vi "SLL DE DO Engine.vi"(8 "error in (no error)":errorcluster) -> (0 "error out":errorcluster)   [LabVIEW 2009]
doc: "Copyright © 2005, Soliton Technologies.\nAll rights reserved."
uses:
  Controls/SLL DE DAQ Engine Options.ctl
  Controls/SLL DE DO Response LV2Global Options.ctl
  Controls/SLL DE DAQ Global Elements.ctl
  Controls/SLL DE DAQ Global Options.ctl
  Controls/SLL DE DO Global Options.ctl
  Controls/SLL DE DO Safe Value Global Options.ctl
  Controls/SLL DE DO Command LV2Global Options.ctl
  <vilib>/DAQmx/write.llb/DAQmx Write (Digital Bool 1Line 1Point).vi
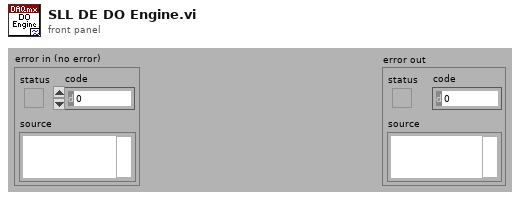
[diagram p1: front panel]
types:
  T1 = typedef "SLL DE DAQ Engine Options.ctl" = enum16{">Init", ">Safe Mode", ">Poll", ">Error", ">Exit", ">Restart", ">DI", ">DO", ">AI", ">AO", ">Start Task", ">Stop Task"}
  T2 = typedef "SLL DE DO Response LV2Global Options.ctl" = enum16{"Initialize", "Send Response", "Check Response", "Close"}
  T3 = cluster{"Previous DO Data":bool[], "Executed for":string, "DO Channels":refnum<k21>[]}
  T4 = typedef "SLL DE DAQ Global Elements.ctl" = enum16{"AI Error", "AO Error", "DI Error", "DO Error", "AI Restart", "DI Restart", "AI Running", "AO Running", "DI Running", "DO Running", "DAQ Exit?"}
  T5 = typedef "SLL DE DAQ Global Options.ctl" = enum16{"Init", "Write 1", "Read 1", "Write Array", "Read Array", "Clear"}
  T6 = typedef "SLL DE DO Global Options.ctl" = enum16{"Init", "Write Line", "Write Array", "Write Full Status", "Read Line", "Read Array", "Read Full Status", "Restart DO", "Send to Safe Mode", "Stop DO"}
  T7 = typedef "SLL DE DO Command LV2Global Options.ctl" = enum16{"Init/Register Events", "Get Event Refnum", "Fire Event", "Destroy Event"}
  T8 = typedef "SLL DE DO Safe Value Global Options.ctl" = enum16{"Read", "Write"}
  T9 = typedef "SLL DE List of Digital Outputs.ctl" = enum16{"STATION1_START TEST", "STATION1_STOP TEST", "STATION1_LIGHT1", "STATION1_LIGHT2", "STATION1_LIGHT3", "STATION2_START TEST", "STATION2_STOP TEST", "STATION2_LIGHT1", "STATION2_LIGHT2", "STATION2_LIGHT3", "STATION3_START TEST", "STATION3_STOP TEST", "STATION3_LIGHT1", "STATION3_LIGHT2", "STATION3_LIGHT3", "STATION4_START TEST", "STATION4_STOP TEST", "STATION4_LIGHT1", "STATION4_LIGHT2", "STATION4_LIGHT3"}
  T10 = enum16{"Left Button", "Center Button", "Right Button", "Window Close"}
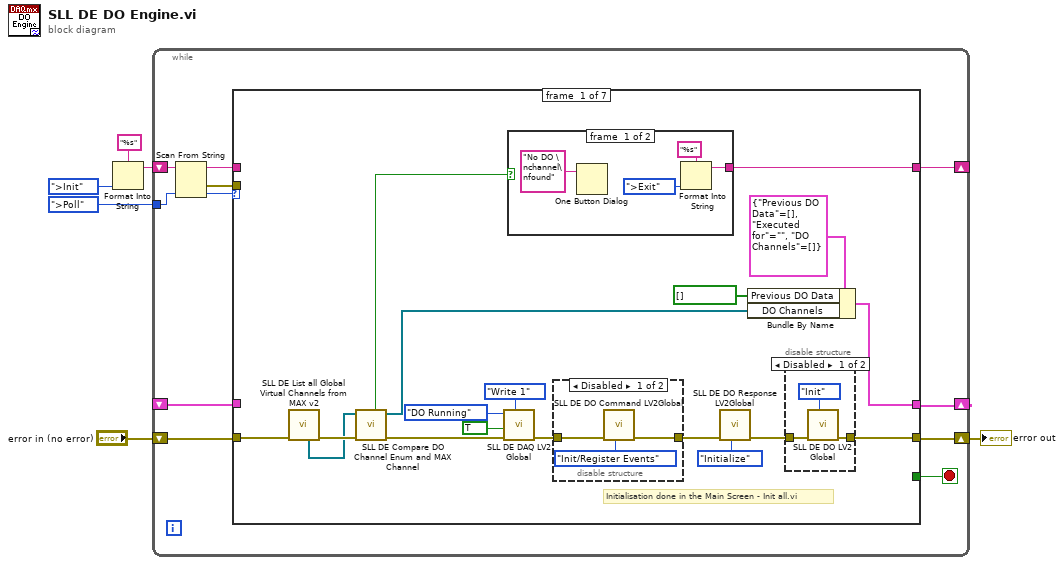
[diagram p0: block diagram]
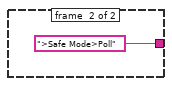
[diagram p4: hidden frame]
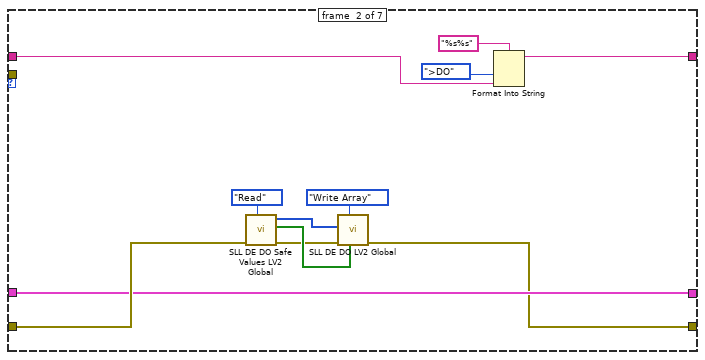
[diagram p5: hidden frame]
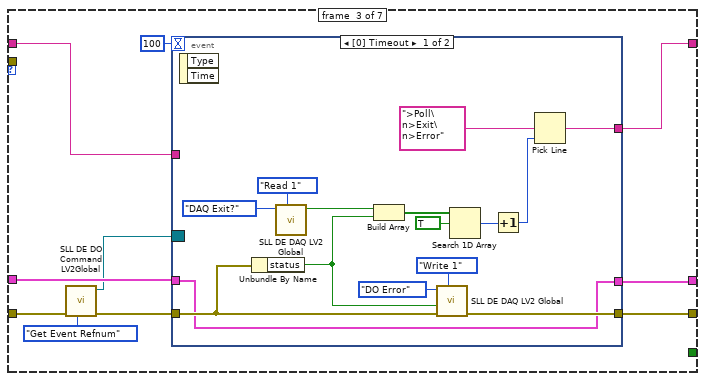
[diagram p6: hidden frame]
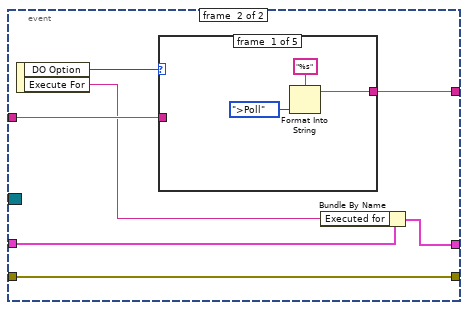
[diagram p7: hidden frame]
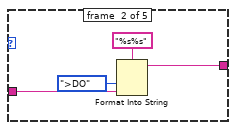
[diagram p8: hidden frame]
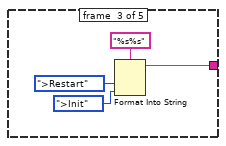
[diagram p9: hidden frame]
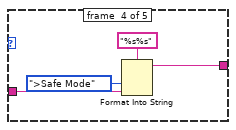
[diagram p10: hidden frame]
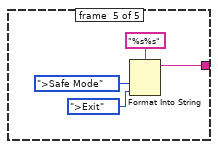
[diagram p11: hidden frame]
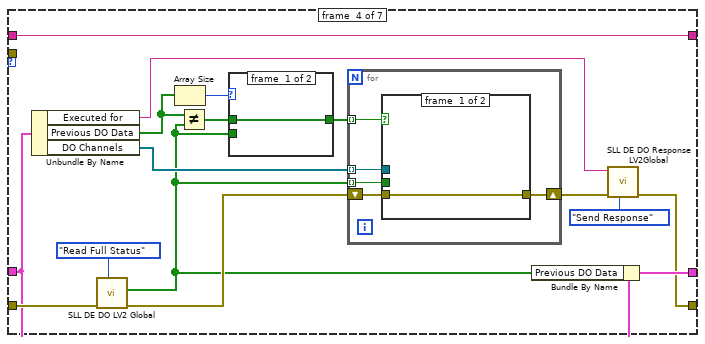
[diagram p12: hidden frame]
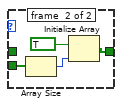
[diagram p13: hidden frame]
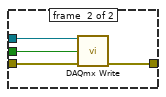
[diagram p14: hidden frame]
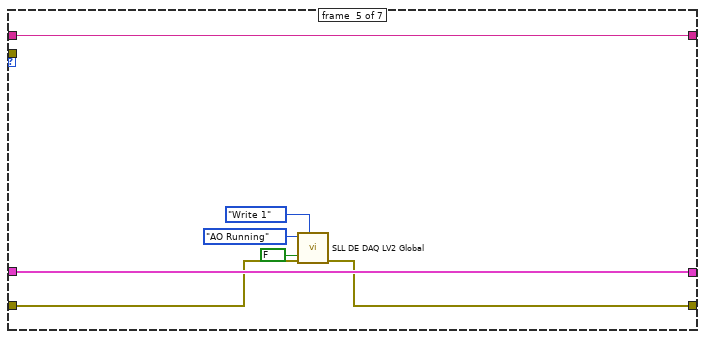
[diagram p15: hidden frame]
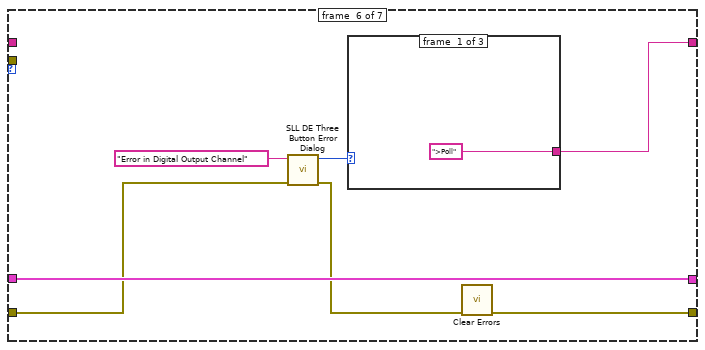
[diagram p16: hidden frame]
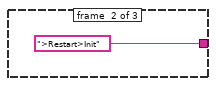
[diagram p17: hidden frame]
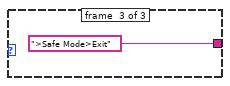
[diagram p18: hidden frame]
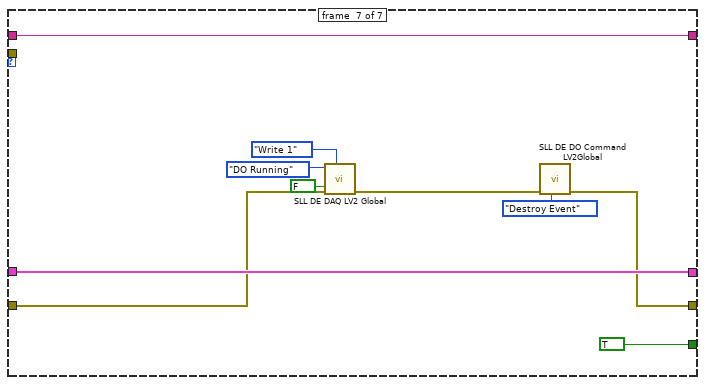
[diagram p19: hidden frame]
diagram:
  n1 = Format Into String(format string="%s", SLL_DE_DAQ_Engine_Options.">Init" ("DAQ Options")) -> (resulting string=w2:string)  [unwired: 2 in, 1 out]
  n2 = while {
    shift-right: [w16] -> w5
    shift-left: "error in (no error)" -> [w17]
    shift-right: [w15] -> _
    shift-left: _ -> [w14]
    shift-right: [w10] -> _
    shift-left: w2 -> [w13]
    tunnel: SLL_DE_DAQ_Engine_Options.">Poll" ("DAQ Options") -> [w7]
    stop <- w9 stop-if-true
    n3 = Scan From String(input string=w13, default 1=w7) -> (remaining string=w12:string, error out=w11:errorcluster, output 1=w8:T1)  [unwired: 3 in, 1 out]
    n4 = case shown="\">Safe Mode\"" w8 {
      tunnel: w17 -> [w28 w57 w67 w125 w144 w154 w163]
      tunnel: [w20 w49 w65 w115 w143 w150 w160] -> w16
      tunnel: [w34 w54 w64 w123 w149 w156 w169] -> w15
      tunnel: w14 -> [_ w54 w66 w112 w149 w156 w169]
      tunnel: w12 -> [_ w52 w62 w124 w148 _ w168]
      tunnel: w11 -> [_ _ _ _ _ _ _]
      tunnel: [w33 w51 w63 w124 w148 w152 w168] -> w10
      tunnel: [_ _ _ _ _ _ TRUE] -> w9
      frame #0 {
        # "Initialisation done in the Main Screen - Init all.vi"
        n5 = call "SLL DE List all Global Virtual Channels from MAX v2.vi"("error in (no error)"=w28) -> ("error out"=w29:errorcluster, "Digital Output"=w26:refnum<k21>[])  [unwired: 4 in, 5 out]
        n6 = call "SLL DE Compare DO Channel Enum and MAX Channel.vi"("error in (no error)"=w29, "Digital Output Channels"=w26) -> ("error out"=w25:errorcluster, "Channels Out"=w19:refnum<k21>[], "Pass?"=w27:bool)  [unwired: 7 in]
        n7 = call "SLL DE DAQ LV2 Global.vi"("Option"=SLL_DE_DAQ_Global_Options."Write 1", "error in (no error)"=w25, "Status In"=TRUE, "Element"=SLL_DE_DAQ_Global_Elements."DO Running") -> ("error out"=w24:errorcluster)  [unwired: 5 in, 2 out]
        n8 = case shown="False" w27 {
          tunnel: [w45 ">Safe Mode>Poll"] -> w33
          frame #0 {
            n9 = One Button Dialog(message="No DO \nchannel\nfound") -> ()  [unwired: 1 in, 1 out]
            n10 = Format Into String(format string="%s", SLL_DE_DAQ_Engine_Options.">Exit" ("DAQ Options")) -> (resulting string=w45:string)  [unwired: 2 in, 1 out]
          }
          frame #1 {
          }
        }
        n11 = disable-structure shown="Disabled" {
          disable-tunnel: w24 -> [w42 w43]
          disable-tunnel: [w40 w43] -> w23
          frame #0 {
            n12 = call "SLL DE DO Command LV2Global.vi"("Option"=SLL_DE_DO_Command_LV2Global_Options."Init/Register Events", "Error in (no error)"=w42) -> ("Error out"=w40:errorcluster)  [unwired: 8 in, 1 out]
          }
          frame #1 {
          }
        }
        n13 = call "SLL DE DO Response LV2Global.vi"("Option"=SLL_DE_DO_Response_LV2Global_Options."Initialize", "Error in (no error)"=w23) -> ("Error out"=w21:errorcluster)  [unwired: 8 in, 1 out]
        n14 = Bundle By Name(cluster=T3 {"Previous DO Data"=[], "Executed for"="", "DO Channels"=[]} ("Data Cluster"), "Previous DO Data"=bool[] [], "DO Channels"=w19) -> (w34:T3)
        n15 = disable-structure shown="Disabled" {
          disable-tunnel: w21 -> [w37 w39]
          disable-tunnel: [w36 w39] -> w20
          frame #0 {
            n16 = call "SLL DE DO LV2 Global.vi"("DO Option"=SLL_DE_DO_Global_Options."Init", "Error In"=w37) -> ("error out"=w36:errorcluster)  [unwired: 6 in, 3 out]
          }
          frame #1 {
          }
        }
      }
      frame #1 {
        n17 = call "SLL DE DO Safe Values LV2 Global.vi"("Cases"=SLL_DE_DO_Safe_Value_Global_Options."Read", "error in (no error)"=w57) -> ("error out"=w58:errorcluster, "Value Array Out"=w59:bool[], "Elements Out"=w60:T9[])  [unwired: 7 in]
        n18 = call "SLL DE DO LV2 Global.vi"("DO State Array"=w59, "DO Option"=SLL_DE_DO_Global_Options."Write Array", "Error In"=w58, "DO Channel Name Array"=w60) -> ("error out"=w49:errorcluster)  [unwired: 4 in, 3 out]
        n19 = Format Into String(format string="%s%s", SLL_DE_DAQ_Engine_Options.">DO" ("DAQ Options"), w52) -> (resulting string=w51:string)  [unwired: 2 in, 1 out]
      }
      frame #2 {
        n20 = call "SLL DE DO Command LV2Global.vi"("Option"=SLL_DE_DO_Command_LV2Global_Options."Get Event Refnum", "Error in (no error)"=w67) -> ("Error out"=w68:errorcluster, "Event Registration Refnum"=w61:refnum<event-registration>)  [unwired: 8 in]
        n21 = event shown="[0] Timeout" {
          selector: w61 -> [_ _]
          dyn-events: _ -> [_ _]
          timeout: 100 -> [_ _]
          tunnel: w68 -> [w76 w91]
          tunnel: [w77 w91] -> w65
          tunnel: [w75 w89] -> w63
          tunnel: w62 -> [_ w90]
          tunnel: w66 -> [w74 w88]
          tunnel: [w74 w86] -> w64
          event #0 {
            n22 = event-data() -> ()  [unwired: 1 in, 2 out]
            n23 = Unbundle By Name(w76) -> ("status"=w85:bool)
            n24 = call "SLL DE DAQ LV2 Global.vi"("Option"=SLL_DE_DAQ_Global_Options."Read 1", "Element"=SLL_DE_DAQ_Global_Elements."DAQ Exit?") -> ("Status Out"=w71:bool)  [unwired: 7 in, 2 out]
            n25 = Build Array(w71, w85) -> (w79:bool[])
            n26 = call "SLL DE DAQ LV2 Global.vi"("Option"=SLL_DE_DAQ_Global_Options."Write 1", "error in (no error)"=w76, "Status In"=w85, "Element"=SLL_DE_DAQ_Global_Elements."DO Error") -> ("error out"=w77:errorcluster)  [unwired: 5 in, 2 out]
            n27 = Search 1D Array(1D array=w79, element=TRUE) -> (index of element=w81:i32)  [unwired: 1 in]
            n28 = Increment(x=w81) -> (x+1=w82:i32)
            n29 = Pick Line(multi-line string=">Poll\n>Exit\n>Error", line index=w82) -> (output string=w75:string)  [unwired: 1 in]
          }
          event #1 {
            n30 = event-data() -> ("DO Option"=w92:T6, "Execute For"=w87:string)  [unwired: 1 in]
            n31 = case shown="\"Init\", Default" w92 {
              tunnel: w90 -> [_ w97 _ w105 _]
              tunnel: [w93 w96 w100 w104 w109] -> w89
              frame #0 {
                n32 = Format Into String(format string="%s", SLL_DE_DAQ_Engine_Options.">Poll" ("DAQ Options")) -> (resulting string=w93:string)  [unwired: 2 in, 1 out]
              }
              frame #1 {
                n33 = Format Into String(format string="%s%s", SLL_DE_DAQ_Engine_Options.">DO" ("DAQ Options"), w97) -> (resulting string=w96:string)  [unwired: 2 in, 1 out]
              }
              frame #2 {
                n34 = Format Into String(format string="%s%s", SLL_DE_DAQ_Engine_Options.">Restart" ("DAQ Options"), SLL_DE_DAQ_Engine_Options.">Init" ("DAQ Options")) -> (resulting string=w100:string)  [unwired: 2 in, 1 out]
              }
              frame #3 {
                n35 = Format Into String(format string="%s%s", SLL_DE_DAQ_Engine_Options.">Safe Mode" ("DAQ Options"), w105) -> (resulting string=w104:string)  [unwired: 2 in, 1 out]
              }
              frame #4 {
                n36 = Format Into String(format string="%s%s", SLL_DE_DAQ_Engine_Options.">Safe Mode" ("DAQ Options"), SLL_DE_DAQ_Engine_Options.">Exit" ("DAQ Options")) -> (resulting string=w109:string)  [unwired: 2 in, 1 out]
              }
            }
            n37 = Bundle By Name(cluster=w88, "Executed for"=w87) -> (w86:T3)
          }
        }
      }
      frame #3 {
        n38 = Unbundle By Name(w112) -> ("Executed for"=w113:string, "Previous DO Data"=w119:bool[], "DO Channels"=w120:refnum<k21>[])
        n39 = call "SLL DE DO LV2 Global.vi"("DO Option"=SLL_DE_DO_Global_Options."Read Full Status", "Error In"=w125) -> ("error out"=w126:errorcluster, "Digital Array Status"=w118:bool[])  [unwired: 6 in, 2 out]
        n40 = Array Size(array=w119) -> (size(s)=w122:i32)
        n41 = Not Equal?(x=w119, y=w118) -> (x != y?=w121:bool[])
        n42 = case shown="0" w122 {
          tunnel: w121 -> [w128 _]
          tunnel: [w128 w131] -> w117
          tunnel: w118 -> [_ w130]
          frame #0 {
          }
          frame #1 {
            n43 = Array Size(array=w130) -> (size(s)=w129:i32)
            n44 = Initialize Array(TRUE, w129) -> (w131:bool[])
          }
        }
        n45 = for {
          tunnel: w117 -> [w137] mode=indexing
          tunnel: w118 -> [w136] mode=indexing
          shift-right: [w134] -> w116
          shift-left: w126 -> [w135]
          tunnel: w120 -> [w133] mode=indexing
          n46 = case shown="True" w137 {
            tunnel: w136 -> [_ w142]
            tunnel: w135 -> [w138 w141]
            tunnel: [w138 w140] -> w134
            tunnel: w133 -> [_ w139]
            frame #0 {
            }
            frame #1 {
              n47 = call-poly <vilib>:"DAQmx Write.vi"("task/channels in"=w139, "data"=w142, "error in"=w141) -> ("error out"=w140:errorcluster)  [unwired: 10 in, 2 out]
            }
          }
        }
        n48 = Bundle By Name(cluster=w112, "Previous DO Data"=w118) -> (w123:T3)
        n49 = call "SLL DE DO Response LV2Global.vi"("Option"=SLL_DE_DO_Response_LV2Global_Options."Send Response", "Error in (no error)"=w116, "Executed For?"=w113) -> ("Error out"=w115:errorcluster)  [unwired: 7 in, 1 out]
      }
      frame #4 {
        n50 = call "SLL DE DAQ LV2 Global.vi"("Option"=SLL_DE_DAQ_Global_Options."Write 1", "error in (no error)"=w144, "Status In"=FALSE, "Element"=SLL_DE_DAQ_Global_Elements."AO Running") -> ("error out"=w143:errorcluster)  [unwired: 5 in, 2 out]
      }
      frame #5 {
        n51 = call "SLL DE Three Button Error Dialog.vi"("Error In"=w154, "Window Title"="Error in Digital Output Channel") -> ("Error Out"=w151:errorcluster, "Which Button?"=w153:T10)  [unwired: 8 in]
        n52 = case shown="\"Center Button\"" w153 {
          tunnel: [">Poll" ("Window Title") ">Restart>Init" ("Window Title") ">Safe Mode>Exit" ("Window Title")] -> w152
          frame #0 {
          }
          frame #1 {
          }
          frame #2 {
          }
        }
        n53 = call <vilib>:"Clear Errors.vi"("error in (no error)"=w151) -> ("error out"=w150:errorcluster)  [unwired: 6 in]
      }
      frame #6 {
        n54 = call "SLL DE DAQ LV2 Global.vi"("Option"=SLL_DE_DAQ_Global_Options."Write 1", "error in (no error)"=w163, "Status In"=FALSE, "Element"=SLL_DE_DAQ_Global_Elements."DO Running") -> ("error out"=w161:errorcluster)  [unwired: 5 in, 2 out]
        n55 = call "SLL DE DO Command LV2Global.vi"("Option"=SLL_DE_DO_Command_LV2Global_Options."Destroy Event", "Error in (no error)"=w161) -> ("Error out"=w160:errorcluster)  [unwired: 8 in, 1 out]
      }
    }
  }
  "error out" <- w5
